vi "Definition.vi"(11 "NewEntityTemplate":refnum<class "Player.lvclass">) -> (2 "Entity Definition":refnum<class "Type.lvclass">[](array[class]))   [LabVIEW 2020, in "Test.lvlib" / "Player.lvclass"]
uses:
  Player.lvclass
  <vilib>/IlluminatedG/IG Conditum Base/Conditum/Columns/Type/Type.lvclass
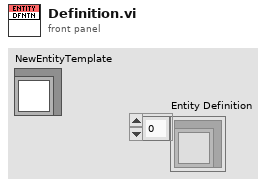
[diagram p1: front panel]
types:
  T1 = typedef "Test.lvlib/Player.lvclass/Columns.ctl" = cluster{"Name":refnum<class "String.lvclass">, "Score":refnum<class "Double.lvclass">, "Active":refnum<class "Boolean.lvclass">}
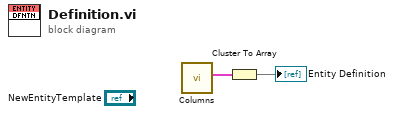
[diagram p0: block diagram]
diagram:
  n1 = call "Columns.vi"() -> ("Columns"=w2:T1)  [unwired: 11 in]
  n2 = Cluster To Array(cluster=w2) -> (array=→"Entity Definition":refnum<class "Type.lvclass">[])
